vi "gato9.vi"() -> ()   [LabVIEW 2015]
doc: "VI principal, manipula los datos para poder pintar sobre la matriz. Tiene dos arreglos, uno de string y otro de color box. Se leerán los valores del array de string para así pintar sobre el array de color box. Para modificar los valores es con los botones."
panel:
  out "error out":errorcluster
  in  "GameOver":bool
  in  "error in (no error)":errorcluster
  in  "9":bool
  in  "8":bool
  in  "7":bool
  in  "6":bool
  in  "5":bool
  in  "4":bool
  in  "3":bool
  in  "2":bool
  in  "1":bool
  in  "Array":u32[][](array[colorbox])
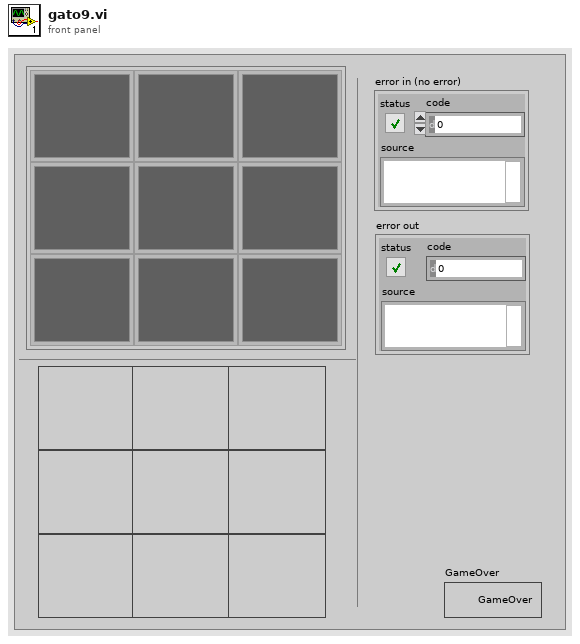
[diagram p1: front panel]
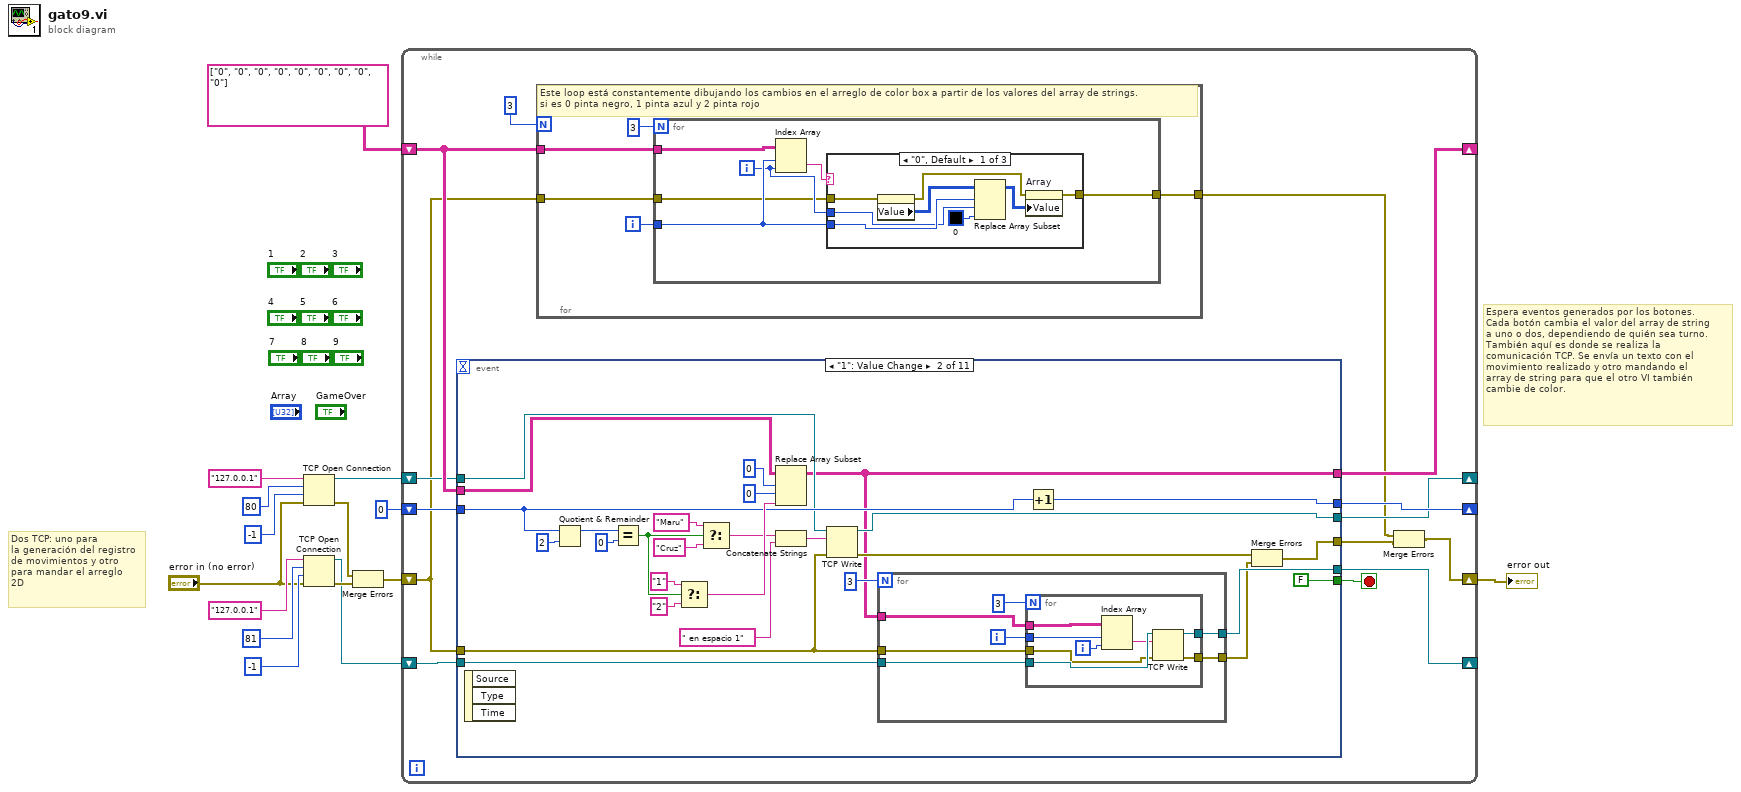
[diagram p0: block diagram]
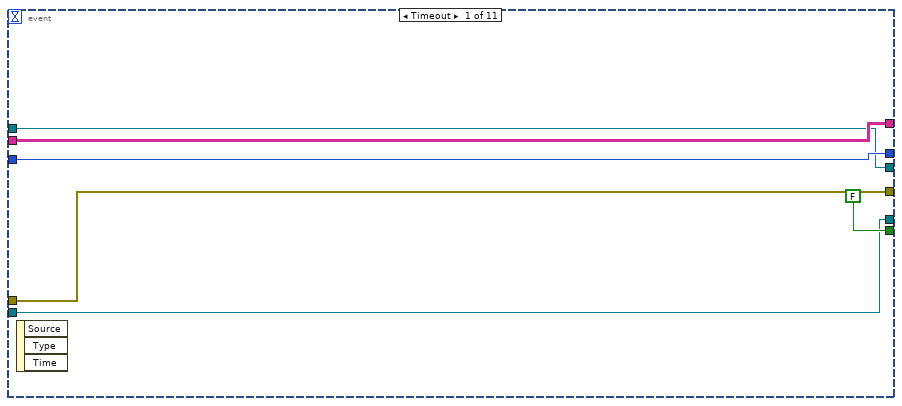
[diagram p2: hidden frame]
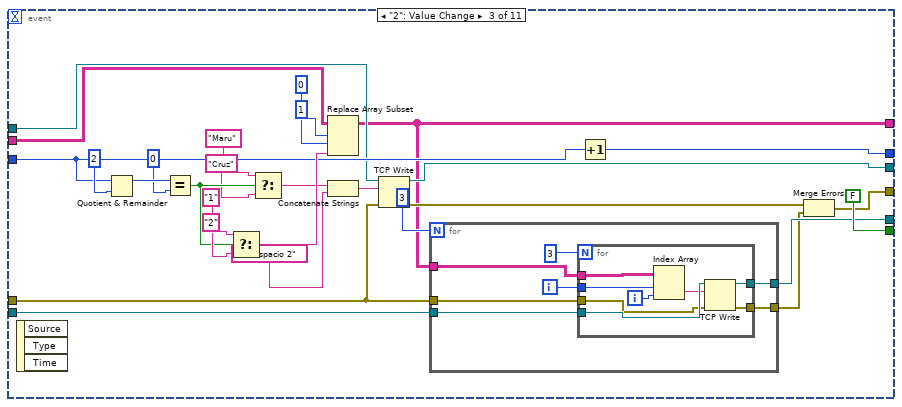
[diagram p3: hidden frame]
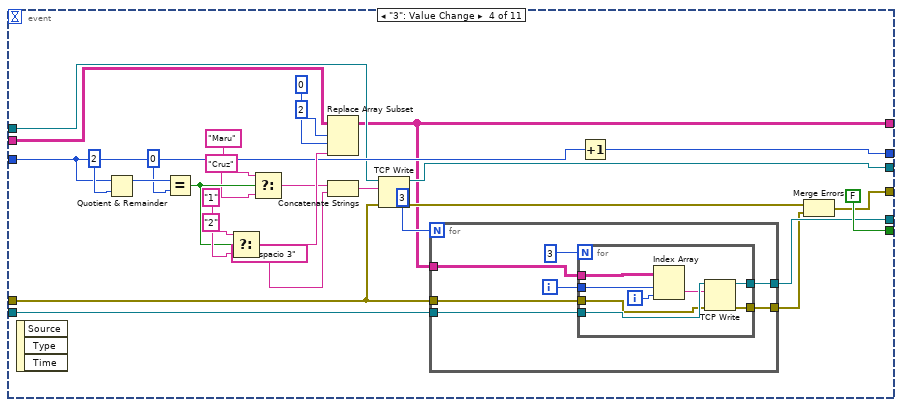
[diagram p4: hidden frame]
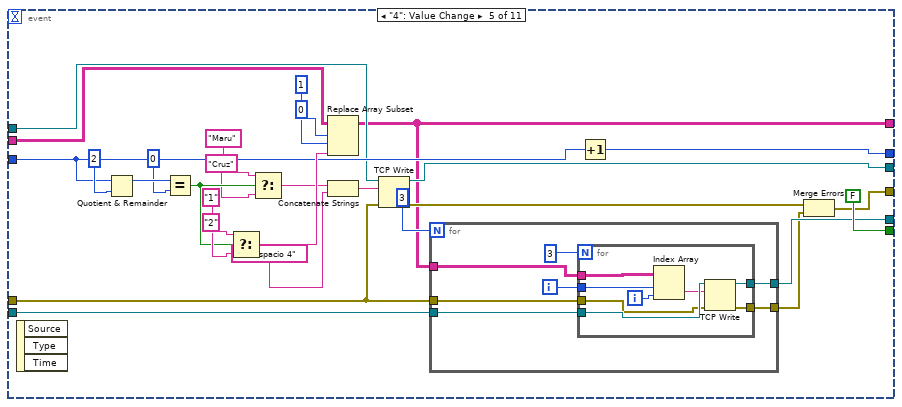
[diagram p5: hidden frame]
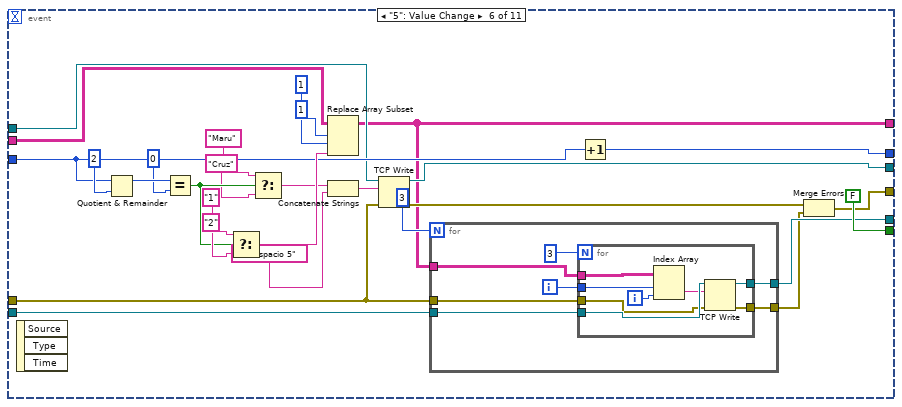
[diagram p6: hidden frame]
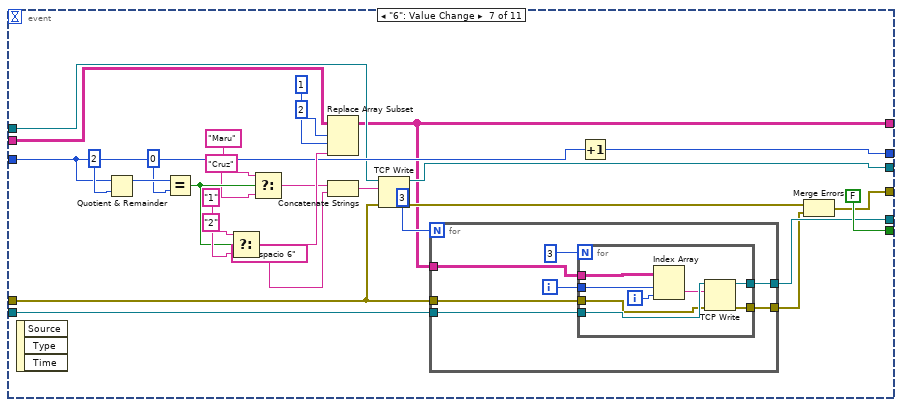
[diagram p7: hidden frame]
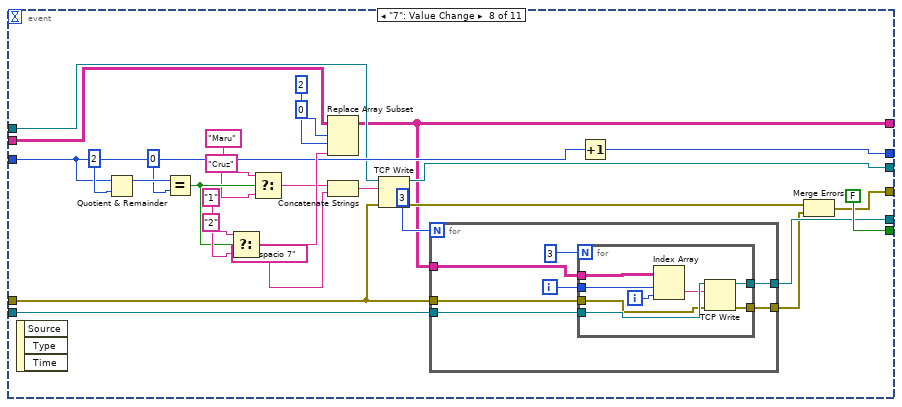
[diagram p8: hidden frame]
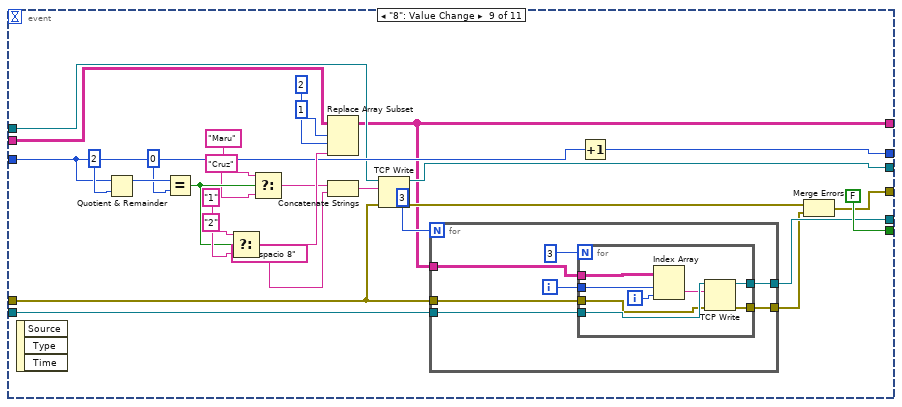
[diagram p9: hidden frame]
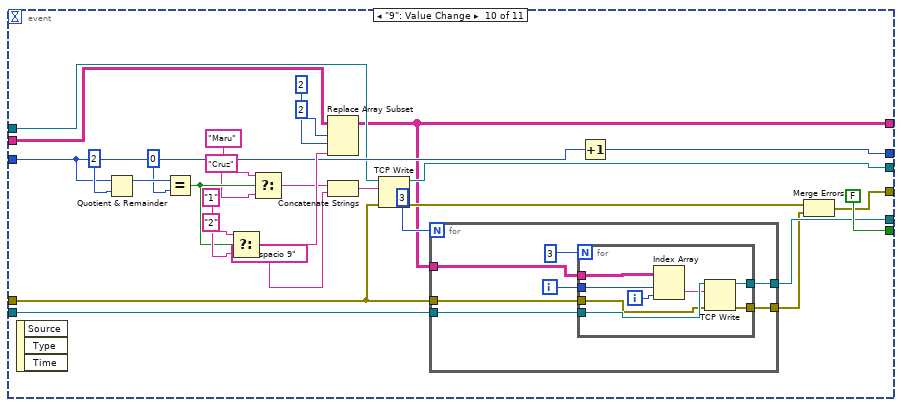
[diagram p10: hidden frame]
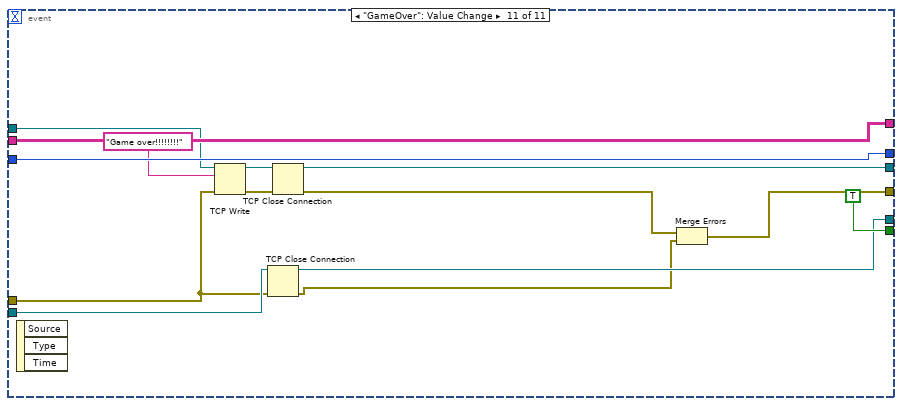
[diagram p11: hidden frame]
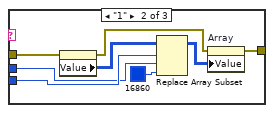
[diagram p12: hidden frame]
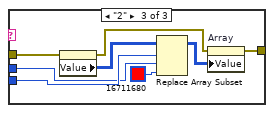
[diagram p13: hidden frame]
diagram:
  # "Espera eventos generados por los botones. \nCada botón cambia el valor del array de string \na uno o dos, dependiendo de quién sea turno. \nTambién aquí es donde se realiza la \ncomunicación TCP. Se envía un texto con el \nmovimiento realizado y otro mandando el \narray de string para que el otro VI también \ncambie de color."
  # "Dos TCP: uno para \nla generación del registro\nde movimientos y otro\npara mandar el arreglo \n2D"
  n1 = TCP Open Connection(address="127.0.0.1" ("IP adress"), remote port or service name=u16 80 ("Port"), timeout ms (60000)=-1 ("timeout ms"), error in (no error)="error in (no error)") -> (connection ID=w10:refnum<k5>, error out=w3:errorcluster)  [unwired: 1 in]
  n2 = TCP Open Connection(address="127.0.0.1" ("IP adress 2"), remote port or service name=u16 81 ("Port 2"), timeout ms (60000)=-1 ("timeout ms  2"), error in (no error)="error in (no error)") -> (connection ID=w1:refnum<k5>, error out=w4:errorcluster)  [unwired: 1 in]
  n3 = Merge Errors(w3, w4) -> (w2:errorcluster)
  n4 = while {
    shift-right: [w28] -> _
    shift-left: string[][] [["0", "0", "0"], ["0", "0", "0"], ["0", "0", "0"]] -> [w27]
    shift-right: [w25] -> _
    shift-left: 0 -> [w26]
    shift-right: [w16] -> w9
    shift-left: w2 -> [w22]
    shift-right: [w21] -> _
    shift-left: w10 -> [w24]
    shift-right: [w19] -> _
    shift-left: w1 -> [w20]
    stop <- w23 stop-if-true
    n5 = event shown="[1] \"1\": Value Change" {
      selector: _ -> [_ _ _ _ _ _ _ _ _ _ _]
      dyn-events: _ -> [_ _ _ _ _ _ _ _ _ _ _]
      timeout: _ -> [_ _ _ _ _ _ _ _ _ _ _]
      tunnel: [w35 w36 w79 w122 w165 w208 w251 w294 w337 w380 w434] -> w28
      tunnel: w27 -> [w35 w42 w85 w128 w171 w214 w257 w300 w343 w386 w434]
      tunnel: w26 -> [w34 w59 w102 w145 w188 w231 w274 w317 w360 w403 w435]
      tunnel: [w34 w58 w101 w144 w187 w230 w273 w316 w359 w402 w435] -> w25
      tunnel: w24 -> [w31 w55 w98 w141 w184 w227 w270 w313 w356 w399 w433]
      tunnel: [FALSE FALSE FALSE FALSE FALSE FALSE FALSE FALSE FALSE FALSE TRUE] -> w23
      tunnel: w22 -> [w32 w38 w81 w124 w167 w210 w253 w296 w339 w382 w426]
      tunnel: [w32 w43 w86 w129 w172 w215 w258 w301 w344 w387 w423] -> w17
      tunnel: [w31 w51 w94 w137 w180 w223 w266 w309 w352 w395 w429] -> w21
      tunnel: w20 -> [w30 w40 w83 w126 w169 w212 w255 w298 w341 w384 w428]
      tunnel: [w30 w39 w82 w125 w168 w211 w254 w297 w340 w383 w427] -> w19
      event Timeout {
        n6 = event-data() -> ()  [unwired: 1 in, 3 out]
      }
      event "1": Value Change {
        n7 = event-data() -> ()  [unwired: 1 in, 3 out]
        n8 = Quotient & Remainder(x=w59, y=2) -> (x-y*floor(x/y)=w62:i32)  [unwired: 1 out]
        n9 = Equal?(x=w62, y=0) -> (x = y?=w50:bool)
        n10 = Select(t="1", s=w50, f="2") -> (s? t:f=w60:string)
        n11 = Select(t="Maru", s=w50, f="Cruz") -> (s? t:f=w47:string)
        n12 = Replace Array Subset(array=w42, new element=w60, index (row)=0, index (col)=0 ("disabled index (col)")) -> (w36:string[][])
        n13 = Concatenate Strings(w47, " en espacio 1") -> (w45:string)
        n14 = TCP Write(connection ID=w55, data in=w45, error in (no error)=w38) -> (connection ID out=w51:refnum<k5>, error out=w44:errorcluster)  [unwired: 1 in, 1 out]
        n15 = for {
          N: 3 -> [_]
          tunnel: w36 -> [w70]
          tunnel: w40 -> [w67]
          tunnel: [w66] -> w39
          tunnel: w38 -> [w65]
          tunnel: [w64] -> w37
          i -> [w69]
          n16 = for {
            N: 3 -> [_]
            tunnel: w70 -> [w78]
            tunnel: w69 -> [w76]
            tunnel: w67 -> [w75]
            tunnel: [w74] -> w66
            tunnel: w65 -> [w72]
            tunnel: [w71] -> w64
            i -> [w77]
            n17 = Index Array(array=w78, index (row)=w76, index (col)=w77) -> (element=w73:string)
            n18 = TCP Write(connection ID=w75, data in=w73, error in (no error)=w72) -> (connection ID out=w74:refnum<k5>, error out=w71:errorcluster)  [unwired: 1 in, 1 out]
          }
        }
        n19 = Increment(x=w59) -> (x+1=w58:i32)
        n20 = Merge Errors(w44, w37) -> (w43:errorcluster)
      }
      event "2": Value Change {
        n21 = event-data() -> ()  [unwired: 1 in, 3 out]
        n22 = Quotient & Remainder(x=w102, y=2) -> (x-y*floor(x/y)=w105:i32)  [unwired: 1 out]
        n23 = Equal?(x=w105, y=0) -> (x = y?=w93:bool)
        n24 = Select(t="1", s=w93, f="2") -> (s? t:f=w103:string)
        n25 = Select(t="Maru", s=w93, f="Cruz") -> (s? t:f=w90:string)
        n26 = Replace Array Subset(array=w85, new element=w103, index (row)=0, index (col)=1 ("disabled index (col)")) -> (w79:string[][])
        n27 = Concatenate Strings(w90, " en espacio 2") -> (w88:string)
        n28 = TCP Write(connection ID=w98, data in=w88, error in (no error)=w81) -> (connection ID out=w94:refnum<k5>, error out=w87:errorcluster)  [unwired: 1 in, 1 out]
        n29 = for {
          N: 3 -> [_]
          tunnel: w79 -> [w113]
          tunnel: w83 -> [w110]
          tunnel: [w109] -> w82
          tunnel: w81 -> [w108]
          tunnel: [w107] -> w80
          i -> [w112]
          n30 = for {
            N: 3 -> [_]
            tunnel: w113 -> [w121]
            tunnel: w112 -> [w119]
            tunnel: w110 -> [w118]
            tunnel: [w117] -> w109
            tunnel: w108 -> [w115]
            tunnel: [w114] -> w107
            i -> [w120]
            n31 = Index Array(array=w121, index (row)=w119, index (col)=w120) -> (element=w116:string)
            n32 = TCP Write(connection ID=w118, data in=w116, error in (no error)=w115) -> (connection ID out=w117:refnum<k5>, error out=w114:errorcluster)  [unwired: 1 in, 1 out]
          }
        }
        n33 = Increment(x=w102) -> (x+1=w101:i32)
        n34 = Merge Errors(w87, w80) -> (w86:errorcluster)
      }
      event "3": Value Change {
        n35 = event-data() -> ()  [unwired: 1 in, 3 out]
        n36 = Quotient & Remainder(x=w145, y=2) -> (x-y*floor(x/y)=w148:i32)  [unwired: 1 out]
        n37 = Equal?(x=w148, y=0) -> (x = y?=w136:bool)
        n38 = Select(t="1", s=w136, f="2") -> (s? t:f=w146:string)
        n39 = Select(t="Maru", s=w136, f="Cruz") -> (s? t:f=w133:string)
        n40 = Replace Array Subset(array=w128, new element=w146, index (row)=0, index (col)=2 ("disabled index (col)")) -> (w122:string[][])
        n41 = Concatenate Strings(w133, " en espacio 3") -> (w131:string)
        n42 = TCP Write(connection ID=w141, data in=w131, error in (no error)=w124) -> (connection ID out=w137:refnum<k5>, error out=w130:errorcluster)  [unwired: 1 in, 1 out]
        n43 = for {
          N: 3 -> [_]
          tunnel: w122 -> [w156]
          tunnel: w126 -> [w153]
          tunnel: [w152] -> w125
          tunnel: w124 -> [w151]
          tunnel: [w150] -> w123
          i -> [w155]
          n44 = for {
            N: 3 -> [_]
            tunnel: w156 -> [w164]
            tunnel: w155 -> [w162]
            tunnel: w153 -> [w161]
            tunnel: [w160] -> w152
            tunnel: w151 -> [w158]
            tunnel: [w157] -> w150
            i -> [w163]
            n45 = Index Array(array=w164, index (row)=w162, index (col)=w163) -> (element=w159:string)
            n46 = TCP Write(connection ID=w161, data in=w159, error in (no error)=w158) -> (connection ID out=w160:refnum<k5>, error out=w157:errorcluster)  [unwired: 1 in, 1 out]
          }
        }
        n47 = Increment(x=w145) -> (x+1=w144:i32)
        n48 = Merge Errors(w130, w123) -> (w129:errorcluster)
      }
      event "4": Value Change {
        n49 = event-data() -> ()  [unwired: 1 in, 3 out]
        n50 = Quotient & Remainder(x=w188, y=2) -> (x-y*floor(x/y)=w191:i32)  [unwired: 1 out]
        n51 = Equal?(x=w191, y=0) -> (x = y?=w179:bool)
        n52 = Select(t="1", s=w179, f="2") -> (s? t:f=w189:string)
        n53 = Select(t="Maru", s=w179, f="Cruz") -> (s? t:f=w176:string)
        n54 = Replace Array Subset(array=w171, new element=w189, index (row)=1, index (col)=0 ("disabled index (col)")) -> (w165:string[][])
        n55 = Concatenate Strings(w176, " en espacio 4") -> (w174:string)
        n56 = TCP Write(connection ID=w184, data in=w174, error in (no error)=w167) -> (connection ID out=w180:refnum<k5>, error out=w173:errorcluster)  [unwired: 1 in, 1 out]
        n57 = for {
          N: 3 -> [_]
          tunnel: w165 -> [w199]
          tunnel: w169 -> [w196]
          tunnel: [w195] -> w168
          tunnel: w167 -> [w194]
          tunnel: [w193] -> w166
          i -> [w198]
          n58 = for {
            N: 3 -> [_]
            tunnel: w199 -> [w207]
            tunnel: w198 -> [w205]
            tunnel: w196 -> [w204]
            tunnel: [w203] -> w195
            tunnel: w194 -> [w201]
            tunnel: [w200] -> w193
            i -> [w206]
            n59 = Index Array(array=w207, index (row)=w205, index (col)=w206) -> (element=w202:string)
            n60 = TCP Write(connection ID=w204, data in=w202, error in (no error)=w201) -> (connection ID out=w203:refnum<k5>, error out=w200:errorcluster)  [unwired: 1 in, 1 out]
          }
        }
        n61 = Increment(x=w188) -> (x+1=w187:i32)
        n62 = Merge Errors(w173, w166) -> (w172:errorcluster)
      }
      event "5": Value Change {
        n63 = event-data() -> ()  [unwired: 1 in, 3 out]
        n64 = Quotient & Remainder(x=w231, y=2) -> (x-y*floor(x/y)=w234:i32)  [unwired: 1 out]
        n65 = Equal?(x=w234, y=0) -> (x = y?=w222:bool)
        n66 = Select(t="1", s=w222, f="2") -> (s? t:f=w232:string)
        n67 = Select(t="Maru", s=w222, f="Cruz") -> (s? t:f=w219:string)
        n68 = Replace Array Subset(array=w214, new element=w232, index (row)=1, index (col)=1 ("disabled index (col)")) -> (w208:string[][])
        n69 = Concatenate Strings(w219, " en espacio 5") -> (w217:string)
        n70 = TCP Write(connection ID=w227, data in=w217, error in (no error)=w210) -> (connection ID out=w223:refnum<k5>, error out=w216:errorcluster)  [unwired: 1 in, 1 out]
        n71 = for {
          N: 3 -> [_]
          tunnel: w208 -> [w242]
          tunnel: w212 -> [w239]
          tunnel: [w238] -> w211
          tunnel: w210 -> [w237]
          tunnel: [w236] -> w209
          i -> [w241]
          n72 = for {
            N: 3 -> [_]
            tunnel: w242 -> [w250]
            tunnel: w241 -> [w248]
            tunnel: w239 -> [w247]
            tunnel: [w246] -> w238
            tunnel: w237 -> [w244]
            tunnel: [w243] -> w236
            i -> [w249]
            n73 = Index Array(array=w250, index (row)=w248, index (col)=w249) -> (element=w245:string)
            n74 = TCP Write(connection ID=w247, data in=w245, error in (no error)=w244) -> (connection ID out=w246:refnum<k5>, error out=w243:errorcluster)  [unwired: 1 in, 1 out]
          }
        }
        n75 = Increment(x=w231) -> (x+1=w230:i32)
        n76 = Merge Errors(w216, w209) -> (w215:errorcluster)
      }
      event "6": Value Change {
        n77 = event-data() -> ()  [unwired: 1 in, 3 out]
        n78 = Quotient & Remainder(x=w274, y=2) -> (x-y*floor(x/y)=w277:i32)  [unwired: 1 out]
        n79 = Equal?(x=w277, y=0) -> (x = y?=w265:bool)
        n80 = Select(t="1", s=w265, f="2") -> (s? t:f=w275:string)
        n81 = Select(t="Maru", s=w265, f="Cruz") -> (s? t:f=w262:string)
        n82 = Replace Array Subset(array=w257, new element=w275, index (row)=1, index (col)=2 ("disabled index (col)")) -> (w251:string[][])
        n83 = Concatenate Strings(w262, " en espacio 6") -> (w260:string)
        n84 = TCP Write(connection ID=w270, data in=w260, error in (no error)=w253) -> (connection ID out=w266:refnum<k5>, error out=w259:errorcluster)  [unwired: 1 in, 1 out]
        n85 = for {
          N: 3 -> [_]
          tunnel: w251 -> [w285]
          tunnel: w255 -> [w282]
          tunnel: [w281] -> w254
          tunnel: w253 -> [w280]
          tunnel: [w279] -> w252
          i -> [w284]
          n86 = for {
            N: 3 -> [_]
            tunnel: w285 -> [w293]
            tunnel: w284 -> [w291]
            tunnel: w282 -> [w290]
            tunnel: [w289] -> w281
            tunnel: w280 -> [w287]
            tunnel: [w286] -> w279
            i -> [w292]
            n87 = Index Array(array=w293, index (row)=w291, index (col)=w292) -> (element=w288:string)
            n88 = TCP Write(connection ID=w290, data in=w288, error in (no error)=w287) -> (connection ID out=w289:refnum<k5>, error out=w286:errorcluster)  [unwired: 1 in, 1 out]
          }
        }
        n89 = Increment(x=w274) -> (x+1=w273:i32)
        n90 = Merge Errors(w259, w252) -> (w258:errorcluster)
      }
      event "7": Value Change {
        n91 = event-data() -> ()  [unwired: 1 in, 3 out]
        n92 = Quotient & Remainder(x=w317, y=2) -> (x-y*floor(x/y)=w320:i32)  [unwired: 1 out]
        n93 = Equal?(x=w320, y=0) -> (x = y?=w308:bool)
        n94 = Select(t="1", s=w308, f="2") -> (s? t:f=w318:string)
        n95 = Select(t="Maru", s=w308, f="Cruz") -> (s? t:f=w305:string)
        n96 = Replace Array Subset(array=w300, new element=w318, index (row)=2, index (col)=0 ("disabled index (col)")) -> (w294:string[][])
        n97 = Concatenate Strings(w305, " en espacio 7") -> (w303:string)
        n98 = TCP Write(connection ID=w313, data in=w303, error in (no error)=w296) -> (connection ID out=w309:refnum<k5>, error out=w302:errorcluster)  [unwired: 1 in, 1 out]
        n99 = for {
          N: 3 -> [_]
          tunnel: w294 -> [w328]
          tunnel: w298 -> [w325]
          tunnel: [w324] -> w297
          tunnel: w296 -> [w323]
          tunnel: [w322] -> w295
          i -> [w327]
          n100 = for {
            N: 3 -> [_]
            tunnel: w328 -> [w336]
            tunnel: w327 -> [w334]
            tunnel: w325 -> [w333]
            tunnel: [w332] -> w324
            tunnel: w323 -> [w330]
            tunnel: [w329] -> w322
            i -> [w335]
            n101 = Index Array(array=w336, index (row)=w334, index (col)=w335) -> (element=w331:string)
            n102 = TCP Write(connection ID=w333, data in=w331, error in (no error)=w330) -> (connection ID out=w332:refnum<k5>, error out=w329:errorcluster)  [unwired: 1 in, 1 out]
          }
        }
        n103 = Increment(x=w317) -> (x+1=w316:i32)
        n104 = Merge Errors(w302, w295) -> (w301:errorcluster)
      }
      event "8": Value Change {
        n105 = event-data() -> ()  [unwired: 1 in, 3 out]
        n106 = Quotient & Remainder(x=w360, y=2) -> (x-y*floor(x/y)=w363:i32)  [unwired: 1 out]
        n107 = Equal?(x=w363, y=0) -> (x = y?=w351:bool)
        n108 = Select(t="1", s=w351, f="2") -> (s? t:f=w361:string)
        n109 = Select(t="Maru", s=w351, f="Cruz") -> (s? t:f=w348:string)
        n110 = Replace Array Subset(array=w343, new element=w361, index (row)=2, index (col)=1 ("disabled index (col)")) -> (w337:string[][])
        n111 = Concatenate Strings(w348, " en espacio 8") -> (w346:string)
        n112 = TCP Write(connection ID=w356, data in=w346, error in (no error)=w339) -> (connection ID out=w352:refnum<k5>, error out=w345:errorcluster)  [unwired: 1 in, 1 out]
        n113 = for {
          N: 3 -> [_]
          tunnel: w337 -> [w371]
          tunnel: w341 -> [w368]
          tunnel: [w367] -> w340
          tunnel: w339 -> [w366]
          tunnel: [w365] -> w338
          i -> [w370]
          n114 = for {
            N: 3 -> [_]
            tunnel: w371 -> [w379]
            tunnel: w370 -> [w377]
            tunnel: w368 -> [w376]
            tunnel: [w375] -> w367
            tunnel: w366 -> [w373]
            tunnel: [w372] -> w365
            i -> [w378]
            n115 = Index Array(array=w379, index (row)=w377, index (col)=w378) -> (element=w374:string)
            n116 = TCP Write(connection ID=w376, data in=w374, error in (no error)=w373) -> (connection ID out=w375:refnum<k5>, error out=w372:errorcluster)  [unwired: 1 in, 1 out]
          }
        }
        n117 = Increment(x=w360) -> (x+1=w359:i32)
        n118 = Merge Errors(w345, w338) -> (w344:errorcluster)
      }
      event "9": Value Change {
        n119 = event-data() -> ()  [unwired: 1 in, 3 out]
        n120 = Quotient & Remainder(x=w403, y=2) -> (x-y*floor(x/y)=w406:i32)  [unwired: 1 out]
        n121 = Equal?(x=w406, y=0) -> (x = y?=w394:bool)
        n122 = Select(t="1", s=w394, f="2") -> (s? t:f=w404:string)
        n123 = Select(t="Maru", s=w394, f="Cruz") -> (s? t:f=w391:string)
        n124 = Replace Array Subset(array=w386, new element=w404, index (row)=2, index (col)=2 ("disabled index (col)")) -> (w380:string[][])
        n125 = Concatenate Strings(w391, " en espacio 9") -> (w389:string)
        n126 = TCP Write(connection ID=w399, data in=w389, error in (no error)=w382) -> (connection ID out=w395:refnum<k5>, error out=w388:errorcluster)  [unwired: 1 in, 1 out]
        n127 = for {
          N: 3 -> [_]
          tunnel: w380 -> [w414]
          tunnel: w384 -> [w411]
          tunnel: [w410] -> w383
          tunnel: w382 -> [w409]
          tunnel: [w408] -> w381
          i -> [w413]
          n128 = for {
            N: 3 -> [_]
            tunnel: w414 -> [w422]
            tunnel: w413 -> [w420]
            tunnel: w411 -> [w419]
            tunnel: [w418] -> w410
            tunnel: w409 -> [w416]
            tunnel: [w415] -> w408
            i -> [w421]
            n129 = Index Array(array=w422, index (row)=w420, index (col)=w421) -> (element=w417:string)
            n130 = TCP Write(connection ID=w419, data in=w417, error in (no error)=w416) -> (connection ID out=w418:refnum<k5>, error out=w415:errorcluster)  [unwired: 1 in, 1 out]
          }
        }
        n131 = Increment(x=w403) -> (x+1=w402:i32)
        n132 = Merge Errors(w388, w381) -> (w387:errorcluster)
      }
      event "GameOver": Value Change {
        n133 = event-data() -> ()  [unwired: 1 in, 3 out]
        n134 = TCP Write(connection ID=w433, data in="Game over!!!!!!!!", error in (no error)=w426) -> (connection ID out=w431:refnum<k5>, error out=w430:errorcluster)  [unwired: 1 in, 1 out]
        n135 = TCP Close Connection(connection ID=w428, error in (no error)=w426) -> (connection ID out=w427:refnum<k5>, error out=w425:errorcluster)  [unwired: 1 in]
        n136 = TCP Close Connection(connection ID=w431, error in (no error)=w430) -> (connection ID out=w429:refnum<k5>, error out=w424:errorcluster)  [unwired: 1 in]
        n137 = Merge Errors(w424, w425) -> (w423:errorcluster)
      }
    }
    n138 = for {
      N: 3 -> [_]
      tunnel: w27 -> [w439]
      tunnel: w22 -> [w438]
      tunnel: [w437] -> w18
      i -> [w441]
      # "Este loop está constantemente dibujando los cambios en el arreglo de color box a partir de los valores del array de strings.\nsi es 0 pinta negro, 1 pinta azul y 2 pinta rojo"
      n139 = for {
        N: 3 -> [_]
        tunnel: w439 -> [w444]
        tunnel: w441 -> [w446]
        tunnel: w438 -> [w443]
        tunnel: [w442] -> w437
        i -> [w445]
        n140 = Index Array(array=w444, index (row)=w446, index (col)=w445) -> (element=w447:string)
        n141 = case shown="\"0\", Default" w447 {
          tunnel: w446 -> [w455 w463 w471]
          tunnel: w445 -> [w453 w461 w469]
          tunnel: w443 -> [w450 w458 w466]
          tunnel: [w448 w456 w464] -> w442
          frame "0", Default {
            n142 = property class="Arr (strict)"(error in=w450) -> (error out=w449:errorcluster, "Value"=w451:u32[][])  [unwired: 1 in, 1 out]
            n143 = Replace Array Subset(array=w451, new element=u32 0, index (row)=w455, index (col)=w453) -> (w454:u32[][])
            n144 = property on="Array" class="Arr (strict)"(error in=w449, "Value"=w454) -> (error out=w448:errorcluster)  [unwired: 1 in, 1 out]
          }
          frame "1" {
            n145 = property class="Arr (strict)"(error in=w458) -> (error out=w457:errorcluster, "Value"=w459:u32[][])  [unwired: 1 in, 1 out]
            n146 = Replace Array Subset(array=w459, new element=u32 16860, index (row)=w463, index (col)=w461) -> (w462:u32[][])
            n147 = property on="Array" class="Arr (strict)"(error in=w457, "Value"=w462) -> (error out=w456:errorcluster)  [unwired: 1 in, 1 out]
          }
          frame "2" {
            n148 = property class="Arr (strict)"(error in=w466) -> (error out=w465:errorcluster, "Value"=w467:u32[][])  [unwired: 1 in, 1 out]
            n149 = Replace Array Subset(array=w467, new element=u32 16711680, index (row)=w471, index (col)=w469) -> (w470:u32[][])
            n150 = property on="Array" class="Arr (strict)"(error in=w465, "Value"=w470) -> (error out=w464:errorcluster)  [unwired: 1 in, 1 out]
          }
        }
      }
    }
    n151 = Merge Errors(w18, w17) -> (w16:errorcluster)
  }
  "error out" <- w9
